vi "sCMOS_main.vi"   [LabVIEW 2015]
uses:
  CONTROLS/Q_camera_element.ctl
  CONTROLS/Q_main_element.ctl
  <vilib>/vision/Image Controls.llb/IMAQ Image.ctl
  CONTROLS/Global parameters.ctl
  GLOBAL/Global_CAMERA.vi
  GLOBAL/Global_ABORT.vi
  GLOBAL/Global_MAIN.vi
types:
  T1 = typedef "Q_main_element.ctl" = cluster{"variant":variant, "Instruction":enum16{"Main_idle", "Main_initialize", "Main_initialize_TDMS", "Main_initialize_Queue", "Main_error", "Main_DAQ_initialization_results", "Main_ASI_initialization_results", "Main_Piezo_initialization_results", "Main_Valve_initialization_results", "Main_Pump_initialization_results", "Main_CAMERA_initialization_results", "Main_FPGA_initialization_results", "Main_DAQ_error", "Main_ASI_error", "Main_Piezo_error", "Main_CAMERA_error", "Main_Valve_error", "Main_Pump_error", "Main_FPGA_error", "Main_start_acquiring", "Main_not_acquiring", "Main_acquiring", "Main_stop_acquiring", "Main_change_exposure", "Main_change_z_scan_parameters", "Main_define_ROI", "Main_define_mosaic", "Main_read_kinetic_time", "Main_cooler", "Main_read_temperature", "Main_save_XY", "Main_load_XY", "Main_discard_XY", "Main_move_to_XY", "Main_measure_QPD", "Main_autofocus_calibration", "Main_autofocus_initialization", "Main_autofocus_stop", "Main_save_PID", "Main_change_H_valve_position", "Main_two_way_valve", "Main_save_movie", "Main_init_single_scan", "Main_single_scan", "Main_stop_single_scan", "Main_merFISH_illumination_parameters", "Main_merFISH_buffer_probe_list", "Main_merFISH_injections_procedure", "Main_merFISH_save_setpoint", "Main_merFISH_DAPI_parameters", "Main_merFISH_Brightfield_parameters", "Main_merFISH_save_embryo_ROI", "Main_merFISH_init", "Main_merFISH_resume", "Main_merFISH_start_autofocus", "Main_merFISH_open_close_valve_merFISH", "Main_merFISH_open_close_valve_photobleaching", "Main_merFISH_hybridization", "Main_merFISH_move_to_ROI", "Main_merFISH_wait_stabilization", "Main_merFISH_move_to_REF", "Main_merFISH_scan", "Main_merFISH_photobleaching_injection", "Main_merFISH_photobleaching", "Main_merFISH_send_email", "Main_merFISH_close", "Main_STOP"}}
  T2 = typedef "Image Type" = u32
  T3 = typedef "Q_camera_element.ctl" = cluster{"variant":variant, "Instruction":enum16{"CAMERA_idle", "CAMERA_initialize", "CAMERA_error", "CAMERA_security_stop", "CAMERA_not_acquiring", "CAMERA_acquiring", "CAMERA_start_acquiring", "CAMERA_stop_acquiring", "CAMERA_change_exposure", "CAMERA_define_ROI", "CAMERA_cooler", "CAMERA_acquire_movie", "CAMERA_init_scan", "CAMERA_check_image_scan", "CAMERA_close_scan", "CAMERA_init_merFISH", "CAMERA_start_acquiring_merFISH", "CAMERA_close_scan_merFISH", "CAMERA_close_merFISH", "CAMERA_STOP"}}
  T4 = typedef "IMAQ Image.ctl" = refnum<image>
  T5 = cluster{"Total kinetic time (s)":dbl, "temperature":dbl, "coolerStatus":i32, "Error":bool, "Real time image":T4}
  T6 = cluster{"Exposure time":dbl, "Start acquisition":bool}
  T7 = cluster{"Sub Region":cluster{"Horizontal Offset":i32, "Vertical Offset":i32, "Horizontal Size":i32, "Vertical Size":i32}, "Start acquisition":bool}
  T8 = typedef "Global parameters.ctl" = cluster{"405":dbl, "488":dbl, "561":dbl, "641":dbl, "BF":dbl, "X":dbl, "Y":dbl, "Filter list":u16, "Exp time":sgl, "Kinetic time":sgl, "Gain":i32, "Step length (nm)":u32, "Total range (nm)":u32, "Scan illumination\n mode":bool, "Dt (s)":i32, "# repetitions":i32}
  T9 = cluster{"Saving path":path, "Sample name":string, "N frames":i32, "N movies":i32, "Start acquisition":bool, "Global parameters":T8}
  T10 = cluster{"Frames":i32, "Movie path":path, "Start acquisition":bool, "Display?":bool}
  T11 = cluster{"Mode":u32, "Polarity":u32, "Times":u32, "Delay":dbl}
  T12 = cluster{"Total frames":i32, "Start acquisition":bool}
  T13 = cluster{"Movie path":path, "Total # frames":i32, "Display?":bool}
  T14 = enum16{"CAMERA_idle", "CAMERA_initialize", "CAMERA_error", "CAMERA_security_stop", "CAMERA_not_acquiring", "CAMERA_acquiring", "CAMERA_start_acquiring", "CAMERA_stop_acquiring", "CAMERA_change_exposure", "CAMERA_define_ROI", "CAMERA_cooler", "CAMERA_acquire_movie", "CAMERA_init_scan", "CAMERA_check_image_scan", "CAMERA_close_scan", "CAMERA_init_merFISH", "CAMERA_start_acquiring_merFISH", "CAMERA_close_scan_merFISH", "CAMERA_close_merFISH", "CAMERA_STOP"}
  T15 = cluster{"Horizontal Offset":i32, "Vertical Offset":i32, "Horizontal Size":i32, "Vertical Size":i32}
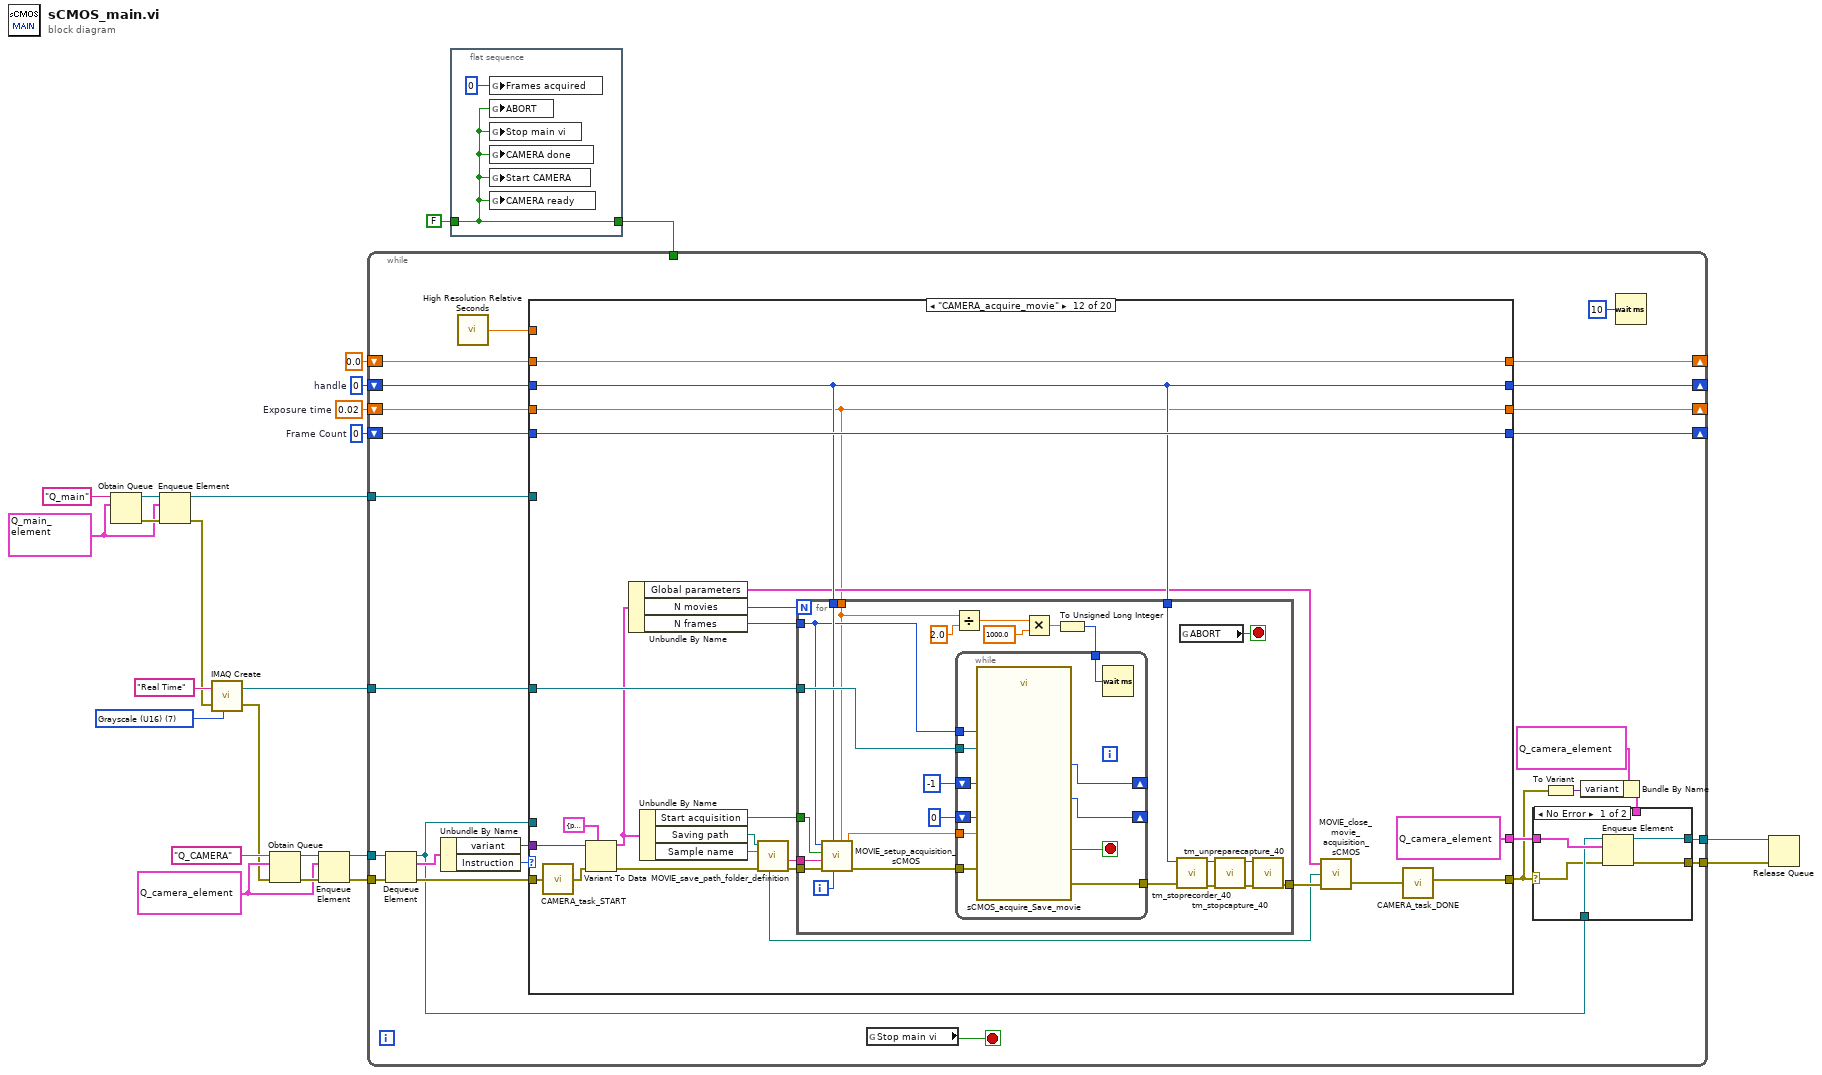
[diagram p0: block diagram]
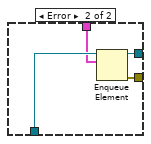
[diagram p2: hidden frame]
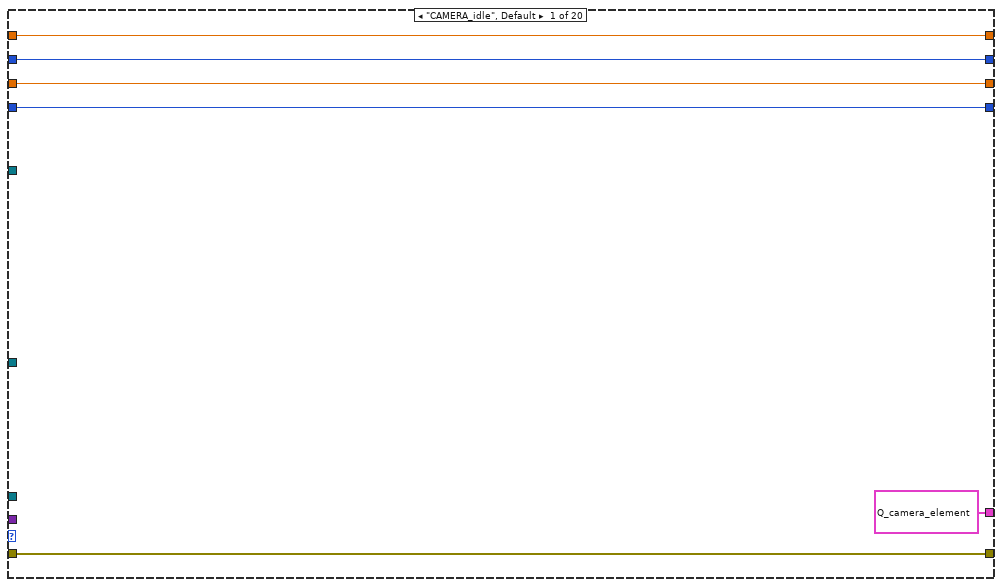
[diagram p3: hidden frame]
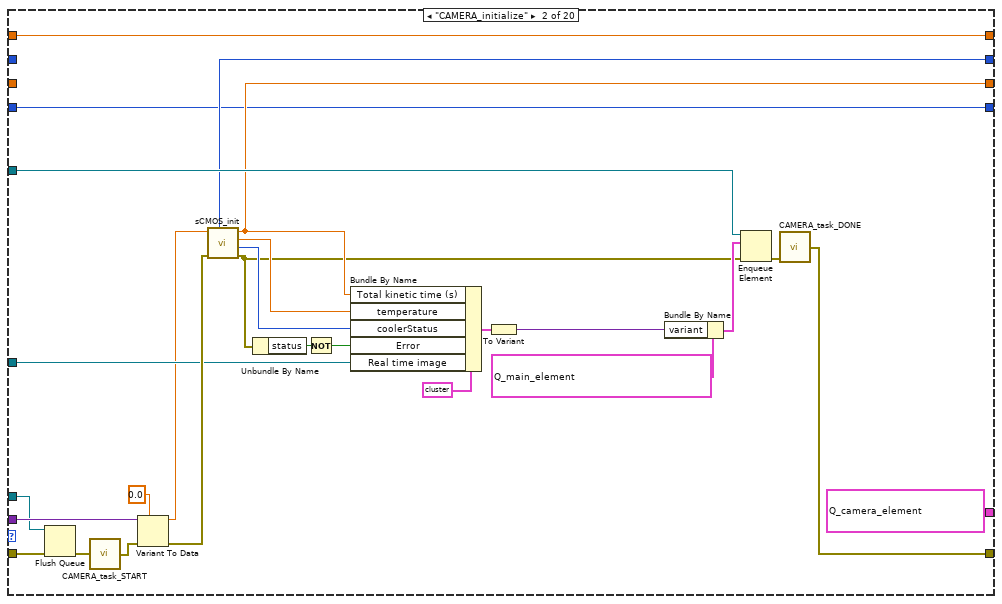
[diagram p4: hidden frame]
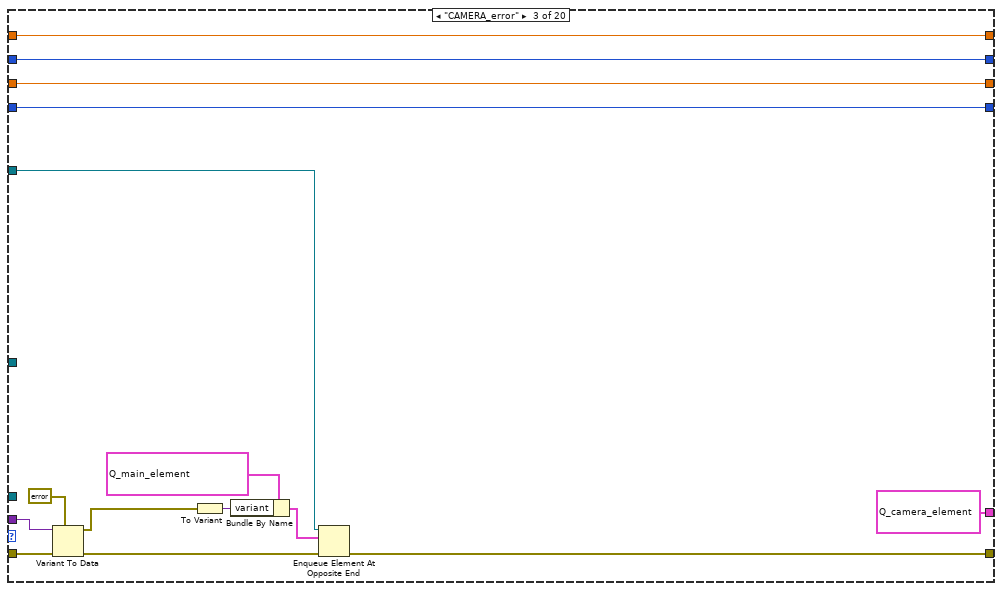
[diagram p5: hidden frame]
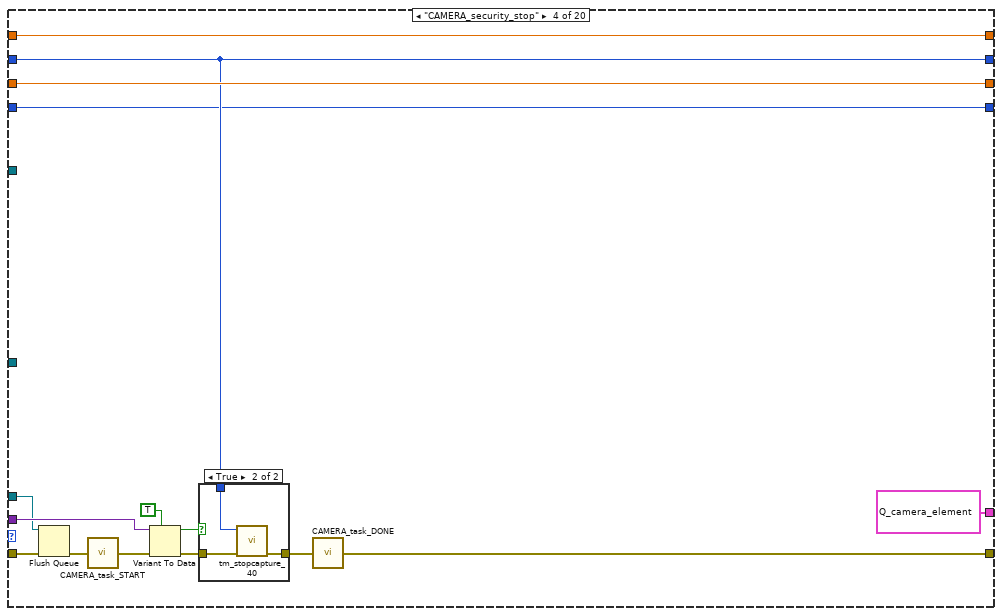
[diagram p6: hidden frame]
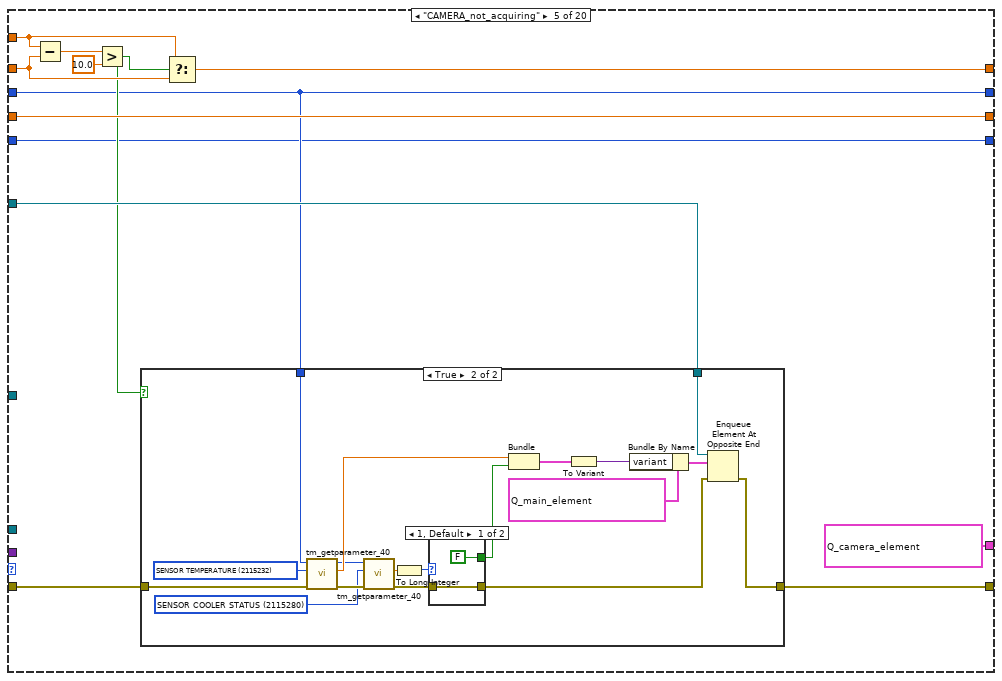
[diagram p8: hidden frame]
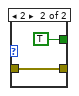
[diagram p10: hidden frame]
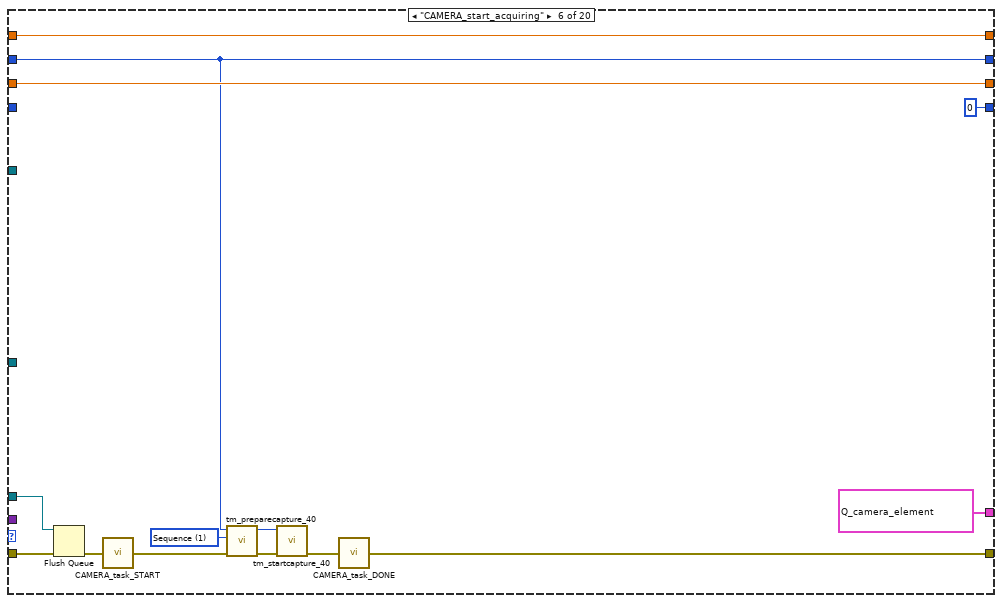
[diagram p11: hidden frame]
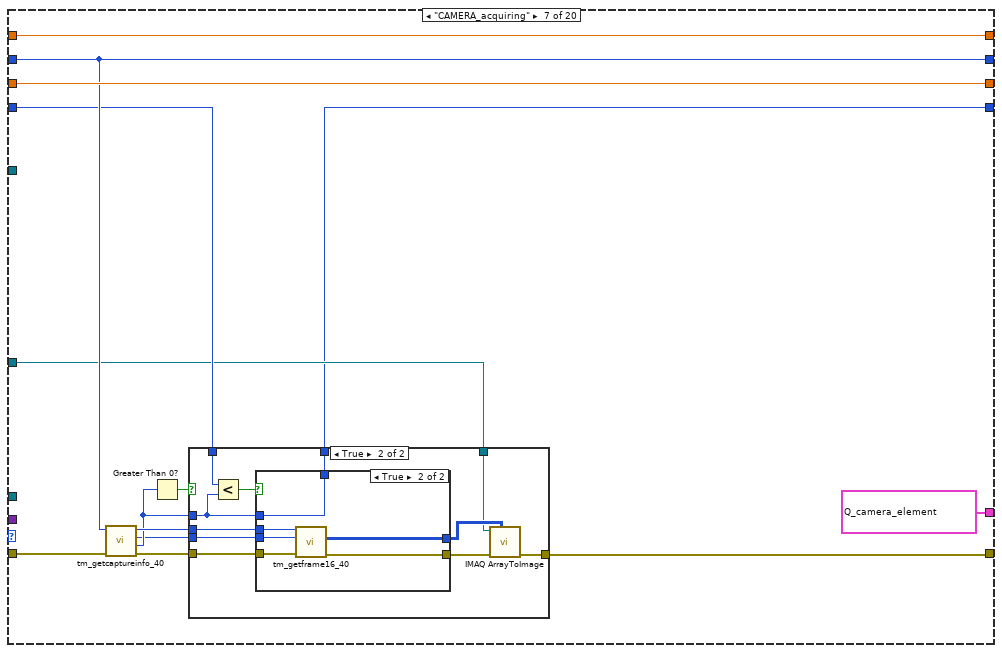
[diagram p12: hidden frame]
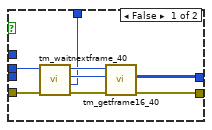
[diagram p14: hidden frame]
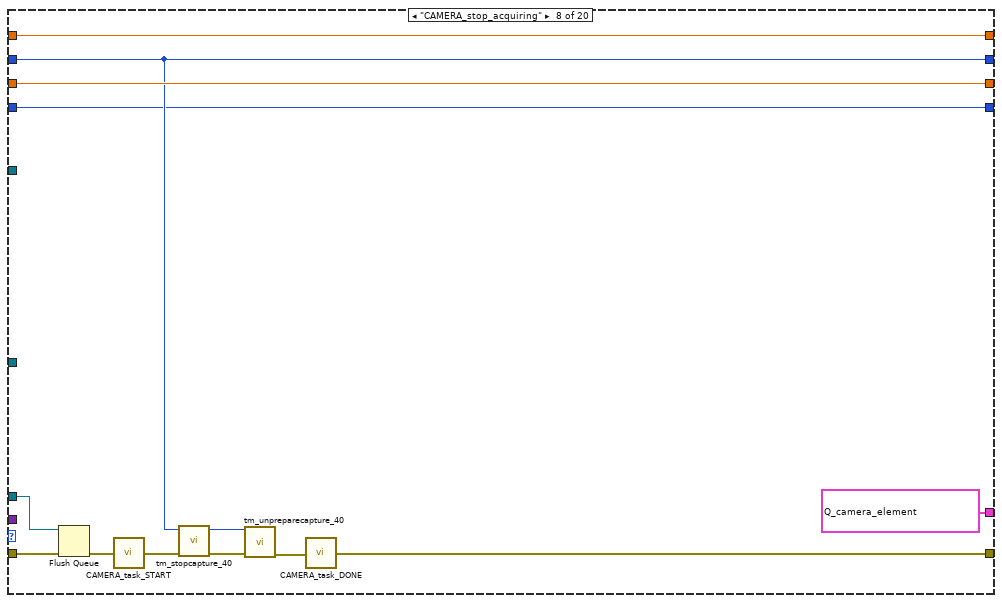
[diagram p15: hidden frame]
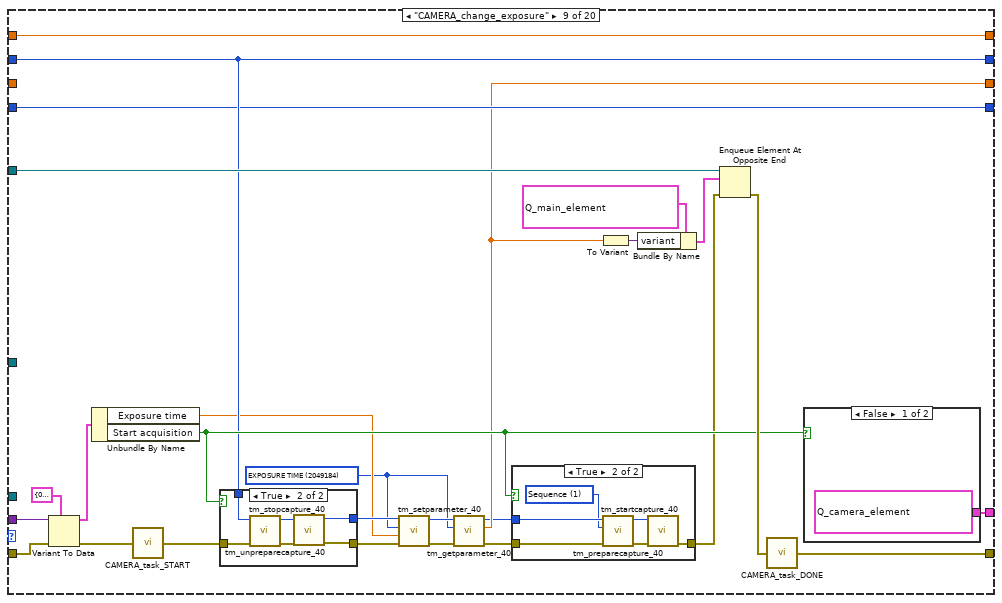
[diagram p16: hidden frame]
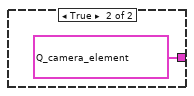
[diagram p18: hidden frame]
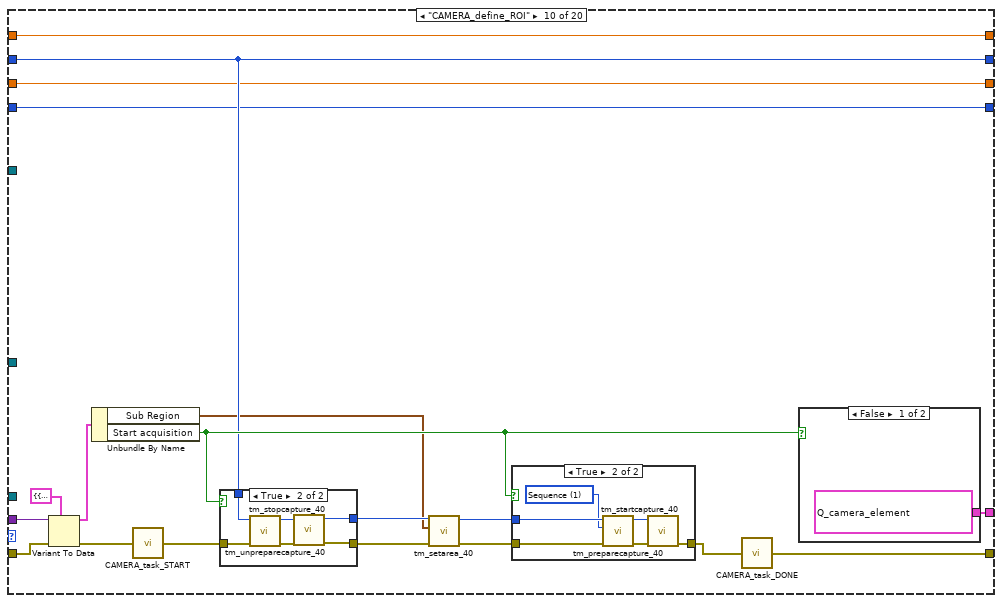
[diagram p20: hidden frame]
diagram:
  w1 = 0  # Frame Count
  w2 = u32 0  # handle
  w3 = T1 {"variant"=variant, "Instruction"=enum."Main_idle"} ("Q_main_element")
  w11 = 0.02  # Exposure time
  w14 = T2 7 items=["Grayscale (U8)", "Grayscale (I16)", "Grayscale (SGL)", "Complex (CSG)", "RGB (U32)", "HSL (U32)", "RGB (U64)", "Grayscale (U16)"] ("Image Type")
  w19 = T3 {"variant"=variant, "Instruction"=enum."CAMERA_idle"} ("Q_ANDOR_element")
  n1 = Obtain Queue(name (unnamed)="Q_main", element data type=w3) -> (queue out=w17:refnum<queue>, error out=w18:errorcluster)  [unwired: 3 in, 1 out]
  n2 = Enqueue Element(queue=w17, element=w3, error in (no error)=w18) -> (queue out=w16:refnum<queue>, error out=w13:errorcluster)  [unwired: 1 in, 1 out]
  n3 = call "IMAQ Create"("Image Name"="Real Time", "Image Type"=w14, "error in (no error)"=w13) -> ("New Image"=w12:T4, "error out"=w9:errorcluster)  [unwired: 2 in]
  n4 = Obtain Queue(name (unnamed)="Q_CAMERA", element data type=w19, error in (no error)=w9) -> (queue out=w23:refnum<queue>, error out=w22:errorcluster)  [unwired: 2 in, 1 out]
  n5 = Enqueue Element(queue=w23, element=w19, error in (no error)=w22) -> (queue out=w21:refnum<queue>, error out=w20:errorcluster)  [unwired: 1 in, 1 out]
  n6 = while {
    tunnel: w21 -> [w50]
    tunnel: w20 -> [w49]
    tunnel: [w44] -> w6
    tunnel: w16 -> [w43]
    tunnel: w12 -> [w41]
    shift-right: [w39] -> _
    shift-left: w11 -> [w40]
    shift-right: [w38] -> _
    shift-left: 0.0 ("Period") -> [w37]
    tunnel: w7 -> [_]
    tunnel: [w36] -> w5
    shift-right: [w30] -> _
    shift-left: w2 -> [w31]
    shift-right: [w28] -> _
    shift-left: w1 -> [w29]
    stop <- w51 stop-if-true
    n7 = Dequeue Element(queue=w50, error in (no error)=w49) -> (queue out=w25:refnum<queue>, element=w48:T3, error out=w46:errorcluster)  [unwired: 1 in, 1 out]
    n8 = Unbundle By Name(w48) -> ("variant"=w42:variant, "Instruction"=w47:T14)
    n9 = call <vilib>:"High Resolution Relative Seconds.vi"() -> ("relative seconds"=w27:dbl)
    n10 = case shown="\"CAMERA_acquire_movie\"" w47 {
      tunnel: w46 -> [w64 w79 w107 w111 w138 w173 w188 w228 w257 w293 w328 w348 w397 w421 w480 w498 w519 w540 w563 w581]
      tunnel: [w64 w75 w94 w120 w137 w174 w180 w227 w250 w289 w323 w346 w406 w420 w481 w497 w522 w541 w564 w579] -> w33
      tunnel: [T3 {"variant"=variant, "Instruction"=enum."CAMERA_idle"} ("Q_ANDOR_element") T3 {"variant"=variant, "Instruction"=enum."CAMERA_not_acquiring"} ("Q_ANDOR_element") T3 {"variant"=variant, "Instruction"=enum."CAMERA_idle"} ("Q_ANDOR_element") T3 {"variant"=variant, "Instruction"=enum."CAMERA_idle"} ("Q_ANDOR_element") T3 {"variant"=variant, "Instruction"=enum."CAMERA_not_acquiring"} ("Q_ANDOR_element") T3 {"variant"=variant, "Instruction"=enum."CAMERA_acquiring"} ("Q_ANDOR_element") T3 {"variant"=variant, "Instruction"=enum."CAMERA_acquiring"} ("Q_ANDOR_element") T3 {"variant"=variant, "Instruction"=enum."CAMERA_not_acquiring"} ("Q_ANDOR_element") w248 w287 T3 {"variant"=variant, "Instruction"=enum."CAMERA_not_acquiring"} ("Q_ANDOR_element") T3 {"variant"=variant, "Instruction"=enum."CAMERA_idle"} ("Q_ANDOR_element") w399 T3 {"variant"=variant, "Instruction"=enum."CAMERA_idle"} ("Q_ANDOR_element") T3 {"variant"=variant, "Instruction"=enum."CAMERA_idle"} ("Q_ANDOR_element") T3 {"variant"=variant, "Instruction"=enum."CAMERA_idle"} ("Q_ANDOR_element") w506 T3 {"variant"=variant, "Instruction"=enum."CAMERA_idle"} ("Q_ANDOR_element") T3 {"variant"=variant, "Instruction"=enum."CAMERA_idle"} ("Q_ANDOR_element") T3 {"variant"=variant, "Instruction"=enum."CAMERA_idle"} ("Q_ANDOR_element")] -> w45
      tunnel: w43 -> [_ w92 w101 _ w134 _ _ _ w253 _ _ _ _ _ _ _ _ _ _ _]
      tunnel: w42 -> [_ w89 w108 w116 _ _ _ _ w258 w294 w327 w352 w407 w427 _ w499 w516 _ _ w571]
      tunnel: w41 -> [_ w83 _ _ _ _ w179 _ _ _ _ w350 _ w426 _ _ _ _ _ w578]
      tunnel: [w65 w76 w97 w121 w139 w177 w191 w230 w234 w283 w325 w329 w404 w424 w478 0.05000000074505806 ("kinetic") w524 w538 w546 w582] -> w39
      tunnel: w40 -> [w65 _ w97 w121 w139 w177 w191 w230 _ w283 w325 w329 w404 w424 w478 _ w524 w538 w546 w582]
      tunnel: w37 -> [w66 w86 w98 w122 w133 w176 w190 w229 w247 w286 w315 w351 w405 w423 w479 w495 w523 w539 w562 w580]
      tunnel: [w66 w86 w98 w122 w131 w176 w190 w229 w247 w286 w315 w351 w405 w423 w479 w495 w523 w539 w562 w580] -> w38
      tunnel: w27 -> [_ _ _ _ w132 _ _ _ _ _ _ _ _ _ _ _ _ _ _ _]
      tunnel: w25 -> [_ w77 _ w109 _ w171 _ w225 _ _ _ _ w395 _ _ w491 w521 _ _ w567]
      tunnel: w31 -> [w62 _ w96 w118 w129 w169 w187 w223 w246 w285 w314 w340 w401 w417 w462 w486 w511 w532 w547 w576]
      tunnel: [w62 w70 w96 w118 w129 w169 w187 w223 w246 w285 w314 w340 w401 w417 w462 w486 w511 w532 w547 w576] -> w30
      tunnel: w29 -> [w61 w69 w95 w117 w128 _ w182 w222 w245 w284 w312 w343 w402 w422 w476 w489 w520 w536 w559 w577]
      tunnel: [w61 w69 w95 w117 w128 0 ("Frame Count") w178 w222 w245 w284 w312 w343 w402 w422 w476 w489 w520 w536 w559 w577] -> w28
      frame "CAMERA_idle", Default {
      }
      frame "CAMERA_initialize" {
        n11 = Flush Queue(queue=w77, error in (no error)=w79) -> (error out=w78:errorcluster)  [unwired: 2 out]
        n12 = call "CAMERA_task_START.vi"("error in"=w78) -> ("error out"=w82:errorcluster)
        n13 = Variant To Data(error in=w82, type=0.0, Variant=w89) -> (data=w73:dbl, error out=w88:errorcluster)
        n14 = call "sCMOS_init.vi"("error in"=w88, "Exposure time"=w73) -> ("error out"=w67:errorcluster, "Cooler status"=w72:i32, "temperature"=w71:dbl, "Exposure time out"=w76:dbl, "Handle out"=w70:u32)  [unwired: 2 in]
        n15 = Unbundle By Name(w67) -> ("status"=w90:bool)
        n16 = Not(x=w90) -> (.not. x?=w87:bool)
        n17 = Bundle By Name(cluster=T5 {"Total kinetic time (s)"=0.0, "temperature"=0.0, "coolerStatus"=0, "Error"=FALSE, "Real time image"=refnum}, "Total kinetic time (s)"=w76, "temperature"=w71, "coolerStatus"=w72, "Error"=w87, "Real time image"=w83) -> (w84:T5)
        n18 = To Variant(anything=w84) -> (Variant=w91:variant)
        n19 = Bundle By Name(cluster=T1 {"variant"=variant, "Instruction"=enum."Main_CAMERA_initialization_results"} ("Q_main_element"), "variant"=w91) -> (w80:T1)
        n20 = Enqueue Element(queue=w92, element=w80, error in (no error)=w67) -> (error out=w68:errorcluster)  [unwired: 1 in, 2 out]
        n21 = call "CAMERA_task_DONE.vi"("error in"=w68) -> ("error out"=w75:errorcluster)
      }
      frame "CAMERA_error" {
        n22 = Variant To Data(error in=w107, type=errorcluster {"status"=FALSE, "code"=0, "source"=""} ("error out"), Variant=w108) -> (data=w103:errorcluster, error out=w100:errorcluster)
        n23 = To Variant(anything=w103) -> (Variant=w104:variant)
        n24 = Bundle By Name(cluster=T1 {"variant"=variant, "Instruction"=enum."Main_CAMERA_error"} ("Q_main_element"), "variant"=w104) -> (w102:T1)
        n25 = Enqueue Element At Opposite End(queue=w101, element=w102, error in (no error)=w100) -> (error out=w94:errorcluster)  [unwired: 1 in, 2 out]
      }
      frame "CAMERA_security_stop" {
        n26 = Flush Queue(queue=w109, error in (no error)=w111) -> (error out=w110:errorcluster)  [unwired: 2 out]
        n27 = call "CAMERA_task_START.vi"("error in"=w110) -> ("error out"=w112:errorcluster)
        n28 = Variant To Data(error in=w112, type=TRUE, Variant=w116) -> (data=w114:bool, error out=w113:errorcluster)
        n29 = case shown="True" w114 {
          tunnel: [w124 w127] -> w119
          tunnel: w118 -> [_ w126]
          tunnel: w113 -> [w124 w125]
          frame False {
          }
          frame True {
            n30 = call <userlib>:"tm_stopcapture_40.vi"("error in (no error)"=w125, "Handle in"=w126) -> ("error out"=w127:errorcluster)  [unwired: 8 in, 1 out]
          }
        }
        n31 = call "CAMERA_task_DONE.vi"("error in"=w119) -> ("error out"=w120:errorcluster)
      }
      frame "CAMERA_not_acquiring" {
        n32 = Subtract(x=w132, y=w133) -> (x-y=w136:dbl)
        n33 = Greater?(x=w136, y=10.0) -> (0:w130:bool)
        n34 = case shown="True" w130 {
          tunnel: w138 -> [w141 w152]
          tunnel: [w141 w159] -> w137
          tunnel: w134 -> [_ w158]
          tunnel: w129 -> [_ w151]
          frame False {
          }
          frame True {
            w146 = u32 2115280 items=["SENSOR MODE"=4212128, "READOUT SPEED"=4211872, "READOUT DIRECTION"=4211904, "TRIGGER GLOBAL EXPOSURE"=2049680, "TRIGGER DELAY"=1066480, "INTERNAL TRIGGER HANDLING"=1066496, "SYNC READOUT SYSTEM BLANK"=1066528, "SENSOR TEMPERATURE"=2115232, "SENSOR COOLER STATUS"=2115280, "EXPOSURE TIME"=2049184, "DEFECT CORRECT MODE"=4670368, "BINNING"=4215968, "INTERNAL LINE SPEED"=4226000, "INTERNAL LINE INTERVAL"=4226016, "NUMBER OF OUTPUT TRIGGER CONNECTOR"=1852320, "OUTPUT TRIGGER SOURCE[0]"=1852576, "OUTPUT TRIGGER SOURCE[1]"=1852832, "OUTPUT TRIGGER SOURCE[2]"=1853088, "OUTPUT TRIGGER POLARITY[0]"=1852592, "OUTPUT TRIGGER POLARITY[1]"=1852848, "OUTPUT TRIGGER POLARITY[2]"=1853104, "OUTPUT TRIGGER ACTIVE[0]"=1852608, "OUTPUT TRIGGER ACTIVE[1]"=1852864, "OUTPUT TRIGGER ACTIVE[2]"=1853120, "OUTPUT TRIGGER DELAY[0]"=1852624, "OUTPUT TRIGGER DELAY[1]"=1852880, "OUTPUT TRIGGER DELAY[2]"=1853136, "OUTPUT TRIGGER PERIOD[0]"=1852640, "OUTPUT TRIGGER PERIOD[1]"=1852896, "OUTPUT TRIGGER PERIOD[2]"=1853152, "OUTPUT TRIGGER KIND[0]"=1852656, "OUTPUT TRIGGER KIND[1]"=1852912, "OUTPUT TRIGGER KIND[2]"=1853168, "OUTPUT TRIGGER BASE SENSOR[0]"=1852672, "OUTPUT TRIGGER BASE SENSOR[1]"=1852928, "OUTPUT TRIGGER BASE SENSOR[2]"=1853184, "OUTPUT TRIGGER PRE HSYNC COUNT"=1852704] ("Parameter")
            w150 = u32 2115232 items=["SENSOR MODE"=4212128, "READOUT SPEED"=4211872, "READOUT DIRECTION"=4211904, "TRIGGER GLOBAL EXPOSURE"=2049680, "TRIGGER DELAY"=1066480, "INTERNAL TRIGGER HANDLING"=1066496, "SYNC READOUT SYSTEM BLANK"=1066528, "SENSOR TEMPERATURE"=2115232, "SENSOR COOLER STATUS"=2115280, "EXPOSURE TIME"=2049184, "DEFECT CORRECT MODE"=4670368, "BINNING"=4215968, "INTERNAL LINE SPEED"=4226000, "INTERNAL LINE INTERVAL"=4226016, "NUMBER OF OUTPUT TRIGGER CONNECTOR"=1852320, "OUTPUT TRIGGER SOURCE[0]"=1852576, "OUTPUT TRIGGER SOURCE[1]"=1852832, "OUTPUT TRIGGER SOURCE[2]"=1853088, "OUTPUT TRIGGER POLARITY[0]"=1852592, "OUTPUT TRIGGER POLARITY[1]"=1852848, "OUTPUT TRIGGER POLARITY[2]"=1853104, "OUTPUT TRIGGER ACTIVE[0]"=1852608, "OUTPUT TRIGGER ACTIVE[1]"=1852864, "OUTPUT TRIGGER ACTIVE[2]"=1853120, "OUTPUT TRIGGER DELAY[0]"=1852624, "OUTPUT TRIGGER DELAY[1]"=1852880, "OUTPUT TRIGGER DELAY[2]"=1853136, "OUTPUT TRIGGER PERIOD[0]"=1852640, "OUTPUT TRIGGER PERIOD[1]"=1852896, "OUTPUT TRIGGER PERIOD[2]"=1853152, "OUTPUT TRIGGER KIND[0]"=1852656, "OUTPUT TRIGGER KIND[1]"=1852912, "OUTPUT TRIGGER KIND[2]"=1853168, "OUTPUT TRIGGER BASE SENSOR[0]"=1852672, "OUTPUT TRIGGER BASE SENSOR[1]"=1852928, "OUTPUT TRIGGER BASE SENSOR[2]"=1853184, "OUTPUT TRIGGER PRE HSYNC COUNT"=1852704] ("Parameter")
            n35 = call <userlib>:"tm_getparameter_40.vi"("error in (no error)"=w152, "Parameter"=w150, "Handle in"=w151) -> ("error out"=w148:errorcluster, "Value out"=w149:dbl, "Handle out"=w147:u32)  [unwired: 6 in]
            n36 = call <userlib>:"tm_getparameter_40.vi"("error in (no error)"=w148, "Parameter"=w146, "Handle in"=w147) -> ("error out"=w144:errorcluster, "Value out"=w145:dbl)  [unwired: 6 in, 1 out]
            n37 = To Long Integer(number=w145) -> (32bit integer=w142:i32)
            n38 = case shown="1, Default" w142 {
              tunnel: [FALSE TRUE] -> w155
              tunnel: w144 -> [w160 w162]
              tunnel: [w160 w162] -> w143
              frame 1, Default {
              }
              frame 2 {
              }
            }
            n39 = Bundle("Value out"=w149, w155) -> (w154:cluster{"Value out":dbl, bool})  [unwired: 1 in]
            n40 = To Variant(anything=w154) -> (Variant=w156:variant)
            n41 = Bundle By Name(cluster=T1 {"variant"=variant, "Instruction"=enum."Main_read_temperature"} ("Q_main_element"), "variant"=w156) -> (w153:T1)
            n42 = Enqueue Element At Opposite End(queue=w158, element=w153, error in (no error)=w143) -> (error out=w159:errorcluster)  [unwired: 1 in, 2 out]
          }
        }
        n43 = Select(t=w132, s=w130, f=w133) -> (s? t:f=w131:dbl)
      }
      frame "CAMERA_start_acquiring" {
        w168 = 1 items=["Snap", "Sequence"] ("Capture mode")
        n44 = Flush Queue(queue=w171, error in (no error)=w173) -> (error out=w172:errorcluster)  [unwired: 2 out]
        n45 = call "CAMERA_task_START.vi"("error in"=w172) -> ("error out"=w170:errorcluster)
        n46 = call <userlib>:"tm_preparecapture_40.vi"("error in (no error)"=w170, "Capture mode"=w168, "Handle in"=w169) -> ("error out"=w167:errorcluster, "Handle out"=w166:u32)  [unwired: 5 in, 2 out]
        n47 = call <userlib>:"tm_startcapture_40.vi"("error in (no error)"=w167, "Handle in"=w166) -> ("error out"=w165:errorcluster)  [unwired: 8 in, 1 out]
        n48 = call "CAMERA_task_DONE.vi"("error in"=w165) -> ("error out"=w174:errorcluster)
      }
      frame "CAMERA_acquiring" {
        n49 = call <userlib>:"tm_getcaptureinfo_40.vi"("error in (no error)"=w188, "Handle in"=w187) -> ("error out"=w184:errorcluster, "Frame Count"=w183:i32, "Frame Index"=w181:i32, "Handle out"=w185:u32)  [unwired: 6 in]
        n50 = Greater Than 0?(x=w183) -> (x > 0?=w186:bool)
        n51 = case shown="True" w186 {
          tunnel: w185 -> [_ w202]
          tunnel: w184 -> [w193 w201]
          tunnel: w183 -> [w192 w194]
          tunnel: w182 -> [_ w204]
          tunnel: w181 -> [_ w200]
          tunnel: [w193 w197] -> w180
          tunnel: w179 -> [_ w196]
          tunnel: [w192 w195] -> w178
          frame False {
          }
          frame True {
            n52 = Less?(x=w204, y=w194) -> (x < y?=w203:bool)
            n53 = case shown="True" w203 {
              tunnel: w202 -> [w211 w218]
              tunnel: w201 -> [w212 w217]
              tunnel: w200 -> [_ w216]
              tunnel: [w206 w215] -> w199
              tunnel: [w207 w214] -> w198
              tunnel: [w205 w213] -> w195
              tunnel: w194 -> [_ w213]
              frame False {
                n54 = call <userlib>:"tm_waitnextframe_40.vi"("error in (no error)"=w212, "Handle in"=w211) -> ("error out"=w210:errorcluster, "Frame Count"=w205:i32, "Frame Index"=w209:i32, "Handle out"=w208:u32)  [unwired: 6 in]
                n55 = call <userlib>:"tm_getframe16_40.vi"("error in (no error)"=w210, "Frame Index"=w209, "Handle in"=w208) -> ("error out"=w206:errorcluster, "Data"=w207:u16[][])  [unwired: 5 in, 2 out]
              }
              frame True {
                n56 = call <userlib>:"tm_getframe16_40.vi"("error in (no error)"=w217, "Frame Index"=w216, "Handle in"=w218) -> ("error out"=w215:errorcluster, "Data"=w214:u16[][])  [unwired: 5 in, 2 out]
              }
            }
            n57 = call "IMAQ ArrayToImage"("Image Pixels (U16)"=w198, "error in (no error)"=w199, "Image"=w196) -> ("error out"=w197:errorcluster)  [unwired: 7 in, 1 out]
          }
        }
      }
      frame "CAMERA_stop_acquiring" {
        n58 = Flush Queue(queue=w225, error in (no error)=w228) -> (error out=w226:errorcluster)  [unwired: 2 out]
        n59 = call "CAMERA_task_START.vi"("error in"=w226) -> ("error out"=w224:errorcluster)
        n60 = call <userlib>:"tm_stopcapture_40.vi"("error in (no error)"=w224, "Handle in"=w223) -> ("error out"=w220:errorcluster, "Handle out"=w221:u32)  [unwired: 8 in]
        n61 = call <userlib>:"tm_unpreparecapture_40.vi"("error in (no error)"=w220, "Handle in"=w221) -> ("error out"=w219:errorcluster)  [unwired: 8 in, 1 out]
        n62 = call "CAMERA_task_DONE.vi"("error in"=w219) -> ("error out"=w227:errorcluster)
      }
      frame "CAMERA_change_exposure" {
        w235 = u32 2049184 items=["SENSOR MODE"=4212128, "READOUT SPEED"=4211872, "READOUT DIRECTION"=4211904, "TRIGGER GLOBAL EXPOSURE"=2049680, "TRIGGER DELAY"=1066480, "INTERNAL TRIGGER HANDLING"=1066496, "SYNC READOUT SYSTEM BLANK"=1066528, "SENSOR TEMPERATURE"=2115232, "SENSOR COOLER STATUS"=2115280, "EXPOSURE TIME"=2049184, "DEFECT CORRECT MODE"=4670368, "BINNING"=4215968, "INTERNAL LINE SPEED"=4226000, "INTERNAL LINE INTERVAL"=4226016, "NUMBER OF OUTPUT TRIGGER CONNECTOR"=1852320, "OUTPUT TRIGGER SOURCE[0]"=1852576, "OUTPUT TRIGGER SOURCE[1]"=1852832, "OUTPUT TRIGGER SOURCE[2]"=1853088, "OUTPUT TRIGGER POLARITY[0]"=1852592, "OUTPUT TRIGGER POLARITY[1]"=1852848, "OUTPUT TRIGGER POLARITY[2]"=1853104, "OUTPUT TRIGGER ACTIVE[0]"=1852608, "OUTPUT TRIGGER ACTIVE[1]"=1852864, "OUTPUT TRIGGER ACTIVE[2]"=1853120, "OUTPUT TRIGGER DELAY[0]"=1852624, "OUTPUT TRIGGER DELAY[1]"=1852880, "OUTPUT TRIGGER DELAY[2]"=1853136, "OUTPUT TRIGGER PERIOD[0]"=1852640, "OUTPUT TRIGGER PERIOD[1]"=1852896, "OUTPUT TRIGGER PERIOD[2]"=1853152, "OUTPUT TRIGGER KIND[0]"=1852656, "OUTPUT TRIGGER KIND[1]"=1852912, "OUTPUT TRIGGER KIND[2]"=1853168, "OUTPUT TRIGGER BASE SENSOR[0]"=1852672, "OUTPUT TRIGGER BASE SENSOR[1]"=1852928, "OUTPUT TRIGGER BASE SENSOR[2]"=1853184, "OUTPUT TRIGGER PRE HSYNC COUNT"=1852704] ("Parameter")
        n63 = Variant To Data(error in=w257, type=T6 {"Exposure time"=0.0, "Start acquisition"=FALSE} ("output cluster"), Variant=w258) -> (data=w254:T6, error out=w256:errorcluster)
        n64 = Unbundle By Name(w254) -> ("Exposure time"=w238:dbl, "Start acquisition"=w249:bool)
        n65 = call "CAMERA_task_START.vi"("error in"=w256) -> ("error out"=w251:errorcluster)
        n66 = case shown="True" w249 {
          tunnel: [w269 w271] -> w240
          tunnel: w251 -> [w269 w275]
          tunnel: w246 -> [w268 w274]
          tunnel: [w268 w270] -> w239
          frame False {
          }
          frame True {
            n67 = call <userlib>:"tm_stopcapture_40.vi"("error in (no error)"=w275, "Handle in"=w274) -> ("error out"=w273:errorcluster, "Handle out"=w272:u32)  [unwired: 8 in]
            n68 = call <userlib>:"tm_unpreparecapture_40.vi"("error in (no error)"=w273, "Handle in"=w272) -> ("error out"=w271:errorcluster, "Handle out"=w270:u32)  [unwired: 8 in]
          }
        }
        n69 = call <userlib>:"tm_setparameter_40.vi"("error in (no error)"=w240, "Value in"=w238, "Parameter"=w235, "Handle in"=w239) -> ("error out"=w237:errorcluster, "Handle out"=w236:u32)  [unwired: 6 in]
        n70 = call <userlib>:"tm_getparameter_40.vi"("error in (no error)"=w237, "Parameter"=w235, "Handle in"=w236) -> ("error out"=w233:errorcluster, "Value out"=w234:dbl, "Handle out"=w232:u32)  [unwired: 6 in]
        n71 = case shown="True" w249 {
          tunnel: w233 -> [w259 w265]
          tunnel: [w259 w260] -> w241
          tunnel: w232 -> [_ w264]
          frame False {
          }
          frame True {
            w263 = 1 items=["Snap", "Sequence"] ("Capture mode")
            n72 = call <userlib>:"tm_preparecapture_40.vi"("error in (no error)"=w265, "Capture mode"=w263, "Handle in"=w264) -> ("error out"=w262:errorcluster, "Handle out"=w261:u32)  [unwired: 5 in, 2 out]
            n73 = call <userlib>:"tm_startcapture_40.vi"("error in (no error)"=w262, "Handle in"=w261) -> ("error out"=w260:errorcluster)  [unwired: 8 in, 1 out]
          }
        }
        n74 = To Variant(anything=w234) -> (Variant=w243:variant)
        n75 = Bundle By Name(cluster=T1 {"variant"=variant, "Instruction"=enum."Main_read_kinetic_time"} ("Q_main_element"), "variant"=w243) -> (w244:T1)
        n76 = Enqueue Element At Opposite End(queue=w253, element=w244, error in (no error)=w241) -> (error out=w252:errorcluster)  [unwired: 1 in, 2 out]
        n77 = call "CAMERA_task_DONE.vi"("error in"=w252) -> ("error out"=w250:errorcluster)
        n78 = case shown="False" w249 {
          tunnel: [T3 {"variant"=variant, "Instruction"=enum."CAMERA_not_acquiring"} ("Q_ANDOR_element") T3 {"variant"=variant, "Instruction"=enum."CAMERA_acquiring"} ("Q_ANDOR_element")] -> w248
          frame False {
          }
          frame True {
          }
        }
      }
      frame "CAMERA_define_ROI" {
        n79 = Variant To Data(error in=w293, type=T7 {"Sub Region"={"Horizontal Offset"=0, "Vertical Offset"=0, "Horizontal Size"=0, "Vertical Size"=0}, "Start acquisition"=FALSE} ("output cluster"), Variant=w294) -> (data=w291:T7, error out=w292:errorcluster)
        n80 = Unbundle By Name(w291) -> ("Sub Region"=w276:T15, "Start acquisition"=w288:bool)
        n81 = call "CAMERA_task_START.vi"("error in"=w292) -> ("error out"=w290:errorcluster)
        n82 = case shown="True" w288 {
          tunnel: [w305 w307] -> w280
          tunnel: w290 -> [w305 w311]
          tunnel: w285 -> [w304 w310]
          tunnel: [w304 w306] -> w278
          frame False {
          }
          frame True {
            n83 = call <userlib>:"tm_stopcapture_40.vi"("error in (no error)"=w311, "Handle in"=w310) -> ("error out"=w309:errorcluster, "Handle out"=w308:u32)  [unwired: 8 in]
            n84 = call <userlib>:"tm_unpreparecapture_40.vi"("error in (no error)"=w309, "Handle in"=w308) -> ("error out"=w307:errorcluster, "Handle out"=w306:u32)  [unwired: 8 in]
          }
        }
        n85 = call <userlib>:"tm_setarea_40.vi"("error in (no error)"=w280, "Sub Region"=w276, "Handle in"=w278) -> ("error out"=w279:errorcluster, "Handle out"=w277:u32)  [unwired: 7 in]
        n86 = case shown="True" w288 {
          tunnel: w279 -> [w295 w301]
          tunnel: [w295 w296] -> w282
          tunnel: w277 -> [_ w300]
          frame False {
          }
          frame True {
            w299 = 1 items=["Snap", "Sequence"] ("Capture mode")
            n87 = call <userlib>:"tm_preparecapture_40.vi"("error in (no error)"=w301, "Capture mode"=w299, "Handle in"=w300) -> ("error out"=w298:errorcluster, "Handle out"=w297:u32)  [unwired: 5 in, 2 out]
            n88 = call <userlib>:"tm_startcapture_40.vi"("error in (no error)"=w298, "Handle in"=w297) -> ("error out"=w296:errorcluster)  [unwired: 8 in, 1 out]
          }
        }
        n89 = call "CAMERA_task_DONE.vi"("error in"=w282) -> ("error out"=w289:errorcluster)
        n90 = case shown="False" w288 {
          tunnel: [T3 {"variant"=variant, "Instruction"=enum."CAMERA_not_acquiring"} ("Q_ANDOR_element") T3 {"variant"=variant, "Instruction"=enum."CAMERA_acquiring"} ("Q_ANDOR_element")] -> w287
          frame False {
          }
          frame True {
          }
        }
      }
      frame "CAMERA_cooler" {
        w316 = u32 2115280 items=["SENSOR MODE"=4212128, "READOUT SPEED"=4211872, "READOUT DIRECTION"=4211904, "TRIGGER GLOBAL EXPOSURE"=2049680, "TRIGGER DELAY"=1066480, "INTERNAL TRIGGER HANDLING"=1066496, "SYNC READOUT SYSTEM BLANK"=1066528, "SENSOR TEMPERATURE"=2115232, "SENSOR COOLER STATUS"=2115280, "EXPOSURE TIME"=2049184, "DEFECT CORRECT MODE"=4670368, "BINNING"=4215968, "INTERNAL LINE SPEED"=4226000, "INTERNAL LINE INTERVAL"=4226016, "NUMBER OF OUTPUT TRIGGER CONNECTOR"=1852320, "OUTPUT TRIGGER SOURCE[0]"=1852576, "OUTPUT TRIGGER SOURCE[1]"=1852832, "OUTPUT TRIGGER SOURCE[2]"=1853088, "OUTPUT TRIGGER POLARITY[0]"=1852592, "OUTPUT TRIGGER POLARITY[1]"=1852848, "OUTPUT TRIGGER POLARITY[2]"=1853104, "OUTPUT TRIGGER ACTIVE[0]"=1852608, "OUTPUT TRIGGER ACTIVE[1]"=1852864, "OUTPUT TRIGGER ACTIVE[2]"=1853120, "OUTPUT TRIGGER DELAY[0]"=1852624, "OUTPUT TRIGGER DELAY[1]"=1852880, "OUTPUT TRIGGER DELAY[2]"=1853136, "OUTPUT TRIGGER PERIOD[0]"=1852640, "OUTPUT TRIGGER PERIOD[1]"=1852896, "OUTPUT TRIGGER PERIOD[2]"=1853152, "OUTPUT TRIGGER KIND[0]"=1852656, "OUTPUT TRIGGER KIND[1]"=1852912, "OUTPUT TRIGGER KIND[2]"=1853168, "OUTPUT TRIGGER BASE SENSOR[0]"=1852672, "OUTPUT TRIGGER BASE SENSOR[1]"=1852928, "OUTPUT TRIGGER BASE SENSOR[2]"=1853184, "OUTPUT TRIGGER PRE HSYNC COUNT"=1852704] ("Parameter")
        n91 = call "CAMERA_task_START.vi"("error in"=w328) -> ("error out"=w324:errorcluster)
        n92 = Variant To Data(error in=w324, type=FALSE ("Cooler"), Variant=w327) -> (data=w321:bool, error out=w318:errorcluster)
        n93 = Select(t=1.0, s=w321, f=2.0) -> (s? t:f=w317:dbl)
        n94 = call <userlib>:"tm_setparameter_40.vi"("error in (no error)"=w318, "Value in"=w317, "Parameter"=w316, "Handle in"=w314) -> ("error out"=w313:errorcluster)  [unwired: 6 in, 1 out]
        n95 = call "CAMERA_task_DONE.vi"("error in"=w313) -> ("error out"=w323:errorcluster)
      }
      frame "CAMERA_acquire_movie" {
        n96 = call "CAMERA_task_START.vi"("error in"=w348) -> ("error out"=w332:errorcluster)
        n97 = Variant To Data(error in=w332, type=T9 {"Saving path"=path "", "Sample name"="", "N frames"=0, "N movies"=0, "Start acquisition"=FALSE, "Global parameters"={"405"=0.0, "488"=0.0, "561"=0.0, "641"=0.0, "BF"=0.0, "X"=0.0, "Y"=0.0, "Filter list"=0, "Exp time"=0.0, "Kinetic time"=0.0, "Gain"=0, "Step length (nm)"=0, "Total range (nm)"=0, "Scan illumination\n mode"=FALSE, "Dt (s)"=0, "# repetitions"=0}} ("output cluster"), Variant=w352) -> (data=w338:T9, error out=w336:errorcluster)
        n98 = Unbundle By Name(w338) -> ("Global parameters"=w339:T8, "N movies"=w344:i32, "N frames"=w342:i32)
        n99 = Unbundle By Name(w338) -> ("Start acquisition"=w331:bool, "Saving path"=w335:path, "Sample name"=w333:string)
        n100 = call "MOVIE_save_path_folder_definition.vi"("error in"=w336, "Sample name"=w333, "Path to the saving folder"=w335) -> ("error out"=w337:errorcluster, "Movie folder"=w330:string, "Parameter path"=w334:path)  [unwired: 3 in]
        n101 = for {
          N: w344 -> [_]
          tunnel: w350 -> [w377]
          tunnel: w337 -> [w374]
          tunnel: [w366] -> w349
          tunnel: w340 -> [w373]
          tunnel: w342 -> [w361]
          tunnel: w340 -> [w370]
          tunnel: w330 -> [w363]
          tunnel: w331 -> [w362]
          tunnel: w329 -> [w359]
          i -> [w360]
          stop <- w353 stop-if-true
          n102 = call "MOVIE_setup_acquisition_sCMOS.vi"("Exposure time"=w359, "Movie number"=w360, "Handle in"=w373, "error in"=w374, "Movie folder name"=w363, "Acquiring"=w362, "frames"=w361) -> ("error out"=w365:errorcluster, "t0"=w364:dbl)  [unwired: 3 in]
          n103 = Divide(x=w359, y=2.0) -> (x/y=w356:dbl)
          n104 = Multiply(x=w356, y=1000.0) -> (x*y=w354:dbl)
          n105 = To Unsigned Long Integer(number=w354) -> (unsigned 32bit integer=w357:u32)
          n106 = while {
            tunnel: w365 -> [w388]
            tunnel: [w387] -> w369
            tunnel: w377 -> [w386]
            shift-right: [w382] -> _
            shift-left: -1 ("Frames acquired out") -> [w385]
            shift-right: [w383] -> _
            shift-left: 0 ("N repeat out") -> [w384]
            tunnel: w361 -> [w381]
            tunnel: w364 -> [w380]
            tunnel: w357 -> [w379]
            stop <- w378 stop-if-true
            n107 = call "sCMOS_acquire_Save_movie.vi"("t0"=w380, "Frames acquired"=w385, "N repeat"=w384, "error in"=w388, "Image IN"=w386, "Number of images"=w381) -> ("Stop?"=w378:bool, "Frames acquired out"=w382:i32, "N repeat out"=w383:i32, "error out"=w387:errorcluster)  [unwired: 10 in]
            n108 = Wait (ms)(milliseconds to wait=w379) -> ()  [unwired: 1 out]
          }
          n109 = call <userlib>:"tm_stoprecorder_40.vi"("error in (no error)"=w369, "Handle in"=w370) -> ("error out"=w372:errorcluster, "Handle out"=w371:u32)  [unwired: 8 in]
          n110 = global read "Global_ABORT.vi" "ABORT"() -> (w353:bool)
          n111 = call <userlib>:"tm_stopcapture_40.vi"("error in (no error)"=w372, "Handle in"=w371) -> ("error out"=w367:errorcluster, "Handle out"=w368:u32)  [unwired: 8 in]
          n112 = call <userlib>:"tm_unpreparecapture_40.vi"("error in (no error)"=w367, "Handle in"=w368) -> ("error out"=w366:errorcluster)  [unwired: 8 in, 1 out]
        }
        n113 = call "MOVIE_close_movie_acquisition_sCMOS.vi"("error in"=w349, "parameters path"=w334, "Global parameters"=w339) -> ("error out"=w347:errorcluster)  [unwired: 1 in]
        n114 = call "CAMERA_task_DONE.vi"("error in"=w347) -> ("error out"=w346:errorcluster)
      }
      frame "CAMERA_init_scan" {
        n115 = Flush Queue(queue=w395, error in (no error)=w397) -> (error out=w396:errorcluster)  [unwired: 2 out]
        n116 = call "CAMERA_task_START.vi"("error in"=w396) -> ("error out"=w398:errorcluster)
        n117 = Variant To Data(error in=w398, type=T10 {"Frames"=0, "Movie path"=path "", "Start acquisition"=FALSE, "Display?"=TRUE} ("output cluster"), Variant=w407) -> (data=w393:T10, error out=w403:errorcluster)
        n118 = call "sCMOS_init_ramp_FPGA.vi"("error in"=w403, "data cluster"=w393, "handle"=w401) -> ("error out"=w390:errorcluster, "Ready?"=w400:bool, "Frames"=w392:i32)
        n119 = flat-sequence {
          tunnel: w400 -> [w409]
          tunnel: w390 -> [w408]
          tunnel: [w408] -> w389
          frame #0 {
            n120 = global write "Global_CAMERA.vi" "CAMERA ready"(w409) -> ()
          }
        }
        n121 = call "CAMERA_task_DONE.vi"("error in"=w389) -> ("error out"=w406:errorcluster)
        n122 = Unbundle By Name(w393) -> ("Display?"=w391:bool)
        n123 = case shown="True" w391 {
          tunnel: [T3 {"variant"=variant, "Instruction"=enum."CAMERA_idle"} ("Q_ANDOR_element") w412] -> w399
          tunnel: w392 -> [_ w411]
          frame False {
          }
          frame True {
            n124 = To Variant(anything=w411) -> (Variant=w413:variant)
            n125 = Bundle By Name(cluster=T3 {"variant"=variant, "Instruction"=enum."CAMERA_check_image_scan"} ("Q_ANDOR_element"), "variant"=w413) -> (w412:T3)
          }
        }
      }
      frame "CAMERA_check_image_scan" {
        # "During the scan, at each step an internal software trigger is sent by the camera to the camera. This step is used to initiate the acquisition of a single image. Since the acquisition is not instantaneous, the program is waiting in a while loop and at each iteration it:\n\n- checks whether the new image is acquired\n- the abort control was not activated\n- the time spent in the loop is not too long (three times the expected acquisition time). \n\nIf one of the three possibilities is checked, the while loop is stopped and the program proceeds."
        n126 = Variant To Data(error in=w421, type=0 ("Frames"), Variant=w427) -> (data=w415:i32, error out=w419:errorcluster)
        n127 = for {
          N: w415 -> [_]
          tunnel: w426 -> [w437]
          tunnel: w417 -> [w433]
          tunnel: w419 -> [w431]
          tunnel: [w432] -> w420
          shift-right: [w428] -> _
          shift-left: 0 ("Frame Count") -> [w430]
          tunnel: w417 -> [w429]
          n128 = while {
            tunnel: w431 -> [w457]
            tunnel: [w453] -> w436
            tunnel: [w456] -> w435
            tunnel: w433 -> [w455]
            tunnel: [w454] -> w434
            tunnel: w430 -> [w452]
            tunnel: [w451] -> w428
            stop <- w459 stop-if-true
            n129 = call <userlib>:"tm_getcaptureinfo_40.vi"("error in (no error)"=w457, "Handle in"=w455) -> ("error out"=w456:errorcluster, "Frame Count"=w451:i32, "Frame Index"=w454:i32)  [unwired: 6 in, 1 out]
            n130 = global read "Global_ABORT.vi" "ABORT"() -> (w461:bool)
            n131 = global read "Global_MAIN.vi" "Stop scan"() -> (w450:bool)
            n132 = Greater?(x=w451, y=w452) -> (0:w453:bool)
            n133 = Wait (ms)(milliseconds to wait=u32 5) -> ()  [unwired: 1 out]
            n134 = Build Array(w450, w461, w453) -> (w460:bool[])
            n135 = Or Array Elements(Boolean array=w460) -> (logical OR=w459:bool)
          }
          n136 = case shown="True" w436 {
            tunnel: w435 -> [w439 w447]
            tunnel: w437 -> [_ w444]
            tunnel: [w438 w445] -> w432
            tunnel: w429 -> [_ w443]
            tunnel: w434 -> [_ w442]
            frame False {
              n137 = flat-sequence {
                tunnel: w439 -> [w441]
                tunnel: [w441] -> w438
                frame #0 {
                  n138 = global write "Global_CAMERA.vi" "CAMERA ready"(FALSE ("ANDOR ready")) -> ()
                }
              }
            }
            frame True {
              n139 = call "sCMOS_get_last_image.vi"("Image In"=w444, "Frame Index"=w442, "Error in"=w447, "Handle in"=w443) -> ("image error"=w446:errorcluster)  [unwired: 2 in]
              n140 = flat-sequence {
                tunnel: w446 -> [w449]
                tunnel: [w449] -> w445
                frame #0 {
                  n141 = global write "Global_CAMERA.vi" "CAMERA ready"(TRUE ("ANDOR ready")) -> ()
                }
              }
            }
          }
        }
      }
      frame "CAMERA_close_scan" {
        n142 = call "CAMERA_task_START.vi"("error in"=w480) -> ("error out"=w463:errorcluster)
        n143 = call <userlib>:"tm_stoprecorder_40.vi"("error in (no error)"=w463, "Handle in"=w462) -> ("error out"=w465:errorcluster, "Handle out"=w464:u32)  [unwired: 8 in]
        n144 = call <userlib>:"tm_stopcapture_40.vi"("error in (no error)"=w465, "Handle in"=w464) -> ("error out"=w474:errorcluster, "Handle out"=w475:u32)  [unwired: 8 in]
        n145 = call <userlib>:"tm_unpreparecapture_40.vi"("error in (no error)"=w474, "Handle in"=w475) -> ("error out"=w472:errorcluster, "Handle out"=w473:u32)  [unwired: 8 in]
        n146 = call <userlib>:"tm_setinputtrigger_40.vi"("error in (no error)"=w472, "Parameters"=T11 {"Mode"=1, "Polarity"=1, "Times"=1, "Delay"=0.0}, "Handle in"=w473) -> ("error out"=w469:errorcluster, "Handle out"=w470:u32)  [unwired: 7 in]
        n147 = call <userlib>:"tm_setoutputtrigger_40.vi"("Port"=1, "error in (no error)"=w469, "Type"=cluster{"Mode":u32, "Polarity":u32} {"Mode"=1, "Polarity"=1}, "Handle in"=w470) -> ("error out"=w467:errorcluster)  [unwired: 6 in, 1 out]
        n148 = call "CAMERA_task_DONE.vi"("error in"=w467) -> ("error out"=w481:errorcluster)
      }
      frame "CAMERA_init_merFISH" {
        n149 = call "CAMERA_task_START.vi"("error in"=w498) -> ("error out"=w493:errorcluster)
        n150 = Flush Queue(queue=w491, error in (no error)=w493) -> (error out=w492:errorcluster)  [unwired: 2 out]
        n151 = Variant To Data(error in=w492, type=T12 {"Total frames"=0, "Start acquisition"=FALSE} ("output cluster"), Variant=w499) -> (data=w484:T12, error out=w488:errorcluster)
        n152 = Unbundle By Name(w484) -> ("Total frames"=w483:i32, "Start acquisition"=w482:bool)
        n153 = call "sCMOS_init_merFISH.vi"("error in"=w488, "Start acquisition"=w482, "N Frames"=w483, "handle"=w486) -> ("error out"=w487:errorcluster)  [unwired: 3 in]
        n154 = case shown="No Error" w487 {
          selector: w487 -> [w501 w503]
          tunnel: [w501 w503] -> w496
          frame Error {
            n155 = global write "Global_CAMERA.vi" "CAMERA ready"(FALSE ("ANDOR ready")) -> ()
          }
          frame No Error {
            n156 = global write "Global_CAMERA.vi" "CAMERA ready"(TRUE ("ANDOR ready")) -> ()
          }
        }
        n157 = call "CAMERA_task_DONE.vi"("error in"=w496) -> ("error out"=w497:errorcluster)
      }
      frame "CAMERA_start_acquiring_merFISH" {
        n158 = call "CAMERA_task_START.vi"("error in"=w519) -> ("error out"=w518:errorcluster)
        n159 = Flush Queue(queue=w521, error in (no error)=w518) -> (error out=w517:errorcluster)  [unwired: 2 out]
        n160 = Variant To Data(error in=w517, type=T13 {"Movie path"=path "", "Total # frames"=0, "Display?"=FALSE} ("output cluster"), Variant=w516) -> (data=w509:T13, error out=w515:errorcluster)
        n161 = Unbundle By Name(w509) -> ("Movie path"=w513:path, "Total # frames"=w514:i32)
        n162 = call <userlib>:"tm_startrecorder_40.vi"("error in (no error)"=w515, "frames"=w514, "File"=w513, "Handle in"=w511) -> ("error out"=w504:errorcluster, "Handle out"=w505:u32)  [unwired: 6 in]
        n163 = call <userlib>:"tm_startcapture_40.vi"("error in (no error)"=w504, "Handle in"=w505) -> ("error out"=w512:errorcluster)  [unwired: 8 in, 1 out]
        n164 = call "CAMERA_task_DONE.vi"("error in"=w512) -> ("error out"=w522:errorcluster)
        n165 = Unbundle By Name(w509) -> ("Display?"=w507:bool, "Total # frames"=w508:i32)
        n166 = case shown="True" w507 {
          tunnel: w508 -> [_ w527]
          tunnel: [T3 {"variant"=variant, "Instruction"=enum."CAMERA_idle"} ("Q_ANDOR_element") w526] -> w506
          frame False {
          }
          frame True {
            n167 = To Variant(anything=w527) -> (Variant=w528:variant)
            n168 = Bundle By Name(cluster=T3 {"variant"=variant, "Instruction"=enum."CAMERA_check_image_scan"} ("Q_ANDOR_element"), "variant"=w528) -> (w526:T3)
          }
        }
      }
      frame "CAMERA_close_scan_merFISH" {
        n169 = call "CAMERA_task_START.vi"("error in"=w540) -> ("error out"=w535:errorcluster)
        n170 = call <userlib>:"tm_stoprecorder_40.vi"("error in (no error)"=w535, "Handle in"=w532) -> ("error out"=w534:errorcluster, "Handle out"=w533:u32)  [unwired: 8 in]
        n171 = call <userlib>:"tm_stopcapture_40.vi"("error in (no error)"=w534, "Handle in"=w533) -> ("error out"=w530:errorcluster)  [unwired: 8 in, 1 out]
        n172 = case shown="No Error" w530 {
          selector: w530 -> [w543 w545]
          tunnel: [w543 w545] -> w531
          frame Error {
            n173 = global write "Global_CAMERA.vi" "CAMERA ready"(FALSE ("ANDOR ready")) -> ()
          }
          frame No Error {
            n174 = global write "Global_CAMERA.vi" "CAMERA ready"(FALSE ("ANDOR ready")) -> ()
          }
        }
        n175 = call "CAMERA_task_DONE.vi"("error in"=w531) -> ("error out"=w541:errorcluster)
      }
      frame "CAMERA_close_merFISH" {
        n176 = call "CAMERA_task_START.vi"("error in"=w563) -> ("error out"=w549:errorcluster)
        n177 = call <userlib>:"tm_stopcapture_40.vi"("error in (no error)"=w549, "Handle in"=w547) -> ("error out"=w557:errorcluster, "Handle out"=w558:u32)  [unwired: 8 in]
        n178 = call <userlib>:"tm_unpreparecapture_40.vi"("error in (no error)"=w557, "Handle in"=w558) -> ("error out"=w555:errorcluster, "Handle out"=w556:u32)  [unwired: 8 in]
        n179 = call <userlib>:"tm_setinputtrigger_40.vi"("error in (no error)"=w555, "Parameters"=T11 {"Mode"=1, "Polarity"=1, "Times"=1, "Delay"=0.0}, "Handle in"=w556) -> ("error out"=w552:errorcluster, "Handle out"=w553:u32)  [unwired: 7 in]
        n180 = call <userlib>:"tm_setoutputtrigger_40.vi"("Port"=1, "error in (no error)"=w552, "Type"=cluster{"Mode":u32, "Polarity":u32} {"Mode"=1, "Polarity"=1}, "Handle in"=w553) -> ("error out"=w548:errorcluster)  [unwired: 6 in, 1 out]
        n181 = flat-sequence {
          tunnel: w548 -> [w566]
          tunnel: [w566] -> w560
          frame #0 {
            n182 = global write "Global_CAMERA.vi" "CAMERA ready"(FALSE ("ANDOR ready")) -> ()
          }
        }
        n183 = call "CAMERA_task_DONE.vi"("error in"=w560) -> ("error out"=w564:errorcluster)
      }
      frame "CAMERA_STOP" {
        n184 = call "CAMERA_task_START.vi"("error in"=w581) -> ("error out"=w574:errorcluster)
        n185 = Flush Queue(queue=w567, error in (no error)=w574) -> (error out=w568:errorcluster)  [unwired: 2 out]
        n186 = call "IMAQ Dispose"("Image"=w578, "error in (no error)"=w568) -> ("error out"=w572:errorcluster)  [unwired: 4 in]
        n187 = Variant To Data(error in=w572, type=FALSE, Variant=w571) -> (data=w569:bool, error out=w570:errorcluster)
        n188 = case shown="True" w569 {
          tunnel: w576 -> [w588 w595]
          tunnel: [w590 w593] -> w575
          tunnel: w570 -> [w589 w592]
          frame True {
            n189 = call <userlib>:"tm_stopcapture_40.vi"("error in (no error)"=w589, "Handle in"=w588) -> ("error out"=w587:errorcluster, "Handle out"=w585:u32)  [unwired: 8 in]
            n190 = call <userlib>:"tm_unpreparecapture_40.vi"("error in (no error)"=w587, "Handle in"=w585) -> ("error out"=w586:errorcluster, "Handle out"=w584:u32)  [unwired: 8 in]
            n191 = call <userlib>:"tm_closecamera_40.vi"("error in (no error)"=w586, "Handle in"=w584) -> ("error out"=w591:errorcluster)  [unwired: 9 in]
            n192 = call <userlib>:"tm_deinitialize_40.vi"("error in (no error)"=w591) -> ("error out"=w590:errorcluster)  [unwired: 10 in]
          }
          frame False {
            n193 = call <userlib>:"tm_closecamera_40.vi"("error in (no error)"=w592, "Handle in"=w595) -> ("error out"=w594:errorcluster)  [unwired: 9 in]
            n194 = call <userlib>:"tm_deinitialize_40.vi"("error in (no error)"=w594) -> ("error out"=w593:errorcluster)  [unwired: 10 in]
          }
        }
        n195 = call "CAMERA_task_DONE.vi"("error in"=w575) -> ("error out"=w579:errorcluster)
      }
    }
    n196 = global read "Global_MAIN.vi" "Stop main vi"() -> (w51:bool)
    n197 = To Variant(anything=w33) -> (Variant=w34:variant)
    n198 = Bundle By Name(cluster=T3 {"variant"=variant, "Instruction"=enum."CAMERA_error"} ("Q_ANDOR_element"), "variant"=w34) -> (w32:T3)
    n199 = case shown="No Error" w33 {
      selector: w33 -> [w52 _]
      tunnel: w45 -> [w56 _]
      tunnel: [w55 w60] -> w44
      tunnel: [w54 w59] -> w36
      tunnel: w25 -> [w53 w58]
      tunnel: w32 -> [_ w57]
      frame No Error {
        n200 = Enqueue Element(queue=w53, element=w56, error in (no error)=w52) -> (queue out=w55:refnum<queue>, error out=w54:errorcluster)  [unwired: 1 in, 1 out]
      }
      frame Error {
        n201 = Enqueue Element(queue=w58, element=w57) -> (queue out=w60:refnum<queue>, error out=w59:errorcluster)  [unwired: 2 in, 1 out]
      }
    }
    n202 = Wait (ms)(milliseconds to wait=u32 10) -> ()  [unwired: 1 out]
  }
  n203 = flat-sequence {
    tunnel: FALSE ("Stop main vi") -> [w596]
    tunnel: [w596] -> w7
    frame #0 {
      n204 = global write "Global_CAMERA.vi" "Frames acquired"(0 ("Frames acquired")) -> ()
      n205 = global write "Global_ABORT.vi" "ABORT"(w596) -> ()
      n206 = global write "Global_MAIN.vi" "Stop main vi"(w596) -> ()
      n207 = global write "Global_CAMERA.vi" "CAMERA done"(w596) -> ()
      n208 = global write "Global_CAMERA.vi" "Start CAMERA"(w596) -> ()
      n209 = global write "Global_CAMERA.vi" "CAMERA ready"(w596) -> ()
    }
  }
  n210 = Release Queue(queue=w6, error in (no error)=w5) -> ()  [unwired: 1 in, 3 out]
